vi "resonant.piezo.config.vi"() -> (3 "appended array":dbl[][](array[numeric]))   [LabVIEW 2012]
doc: "SciScan 1.2 160622"
uses:
  GFG/GFGnumericGet.vi
  GFG/GFGbooleanGet.vi
  GFG/GFG library.lvlib
panel:
  out "error out":errorcluster
  out "pockels cell control":dbl[](graph)
  out "piezo control":dbl[](graph)
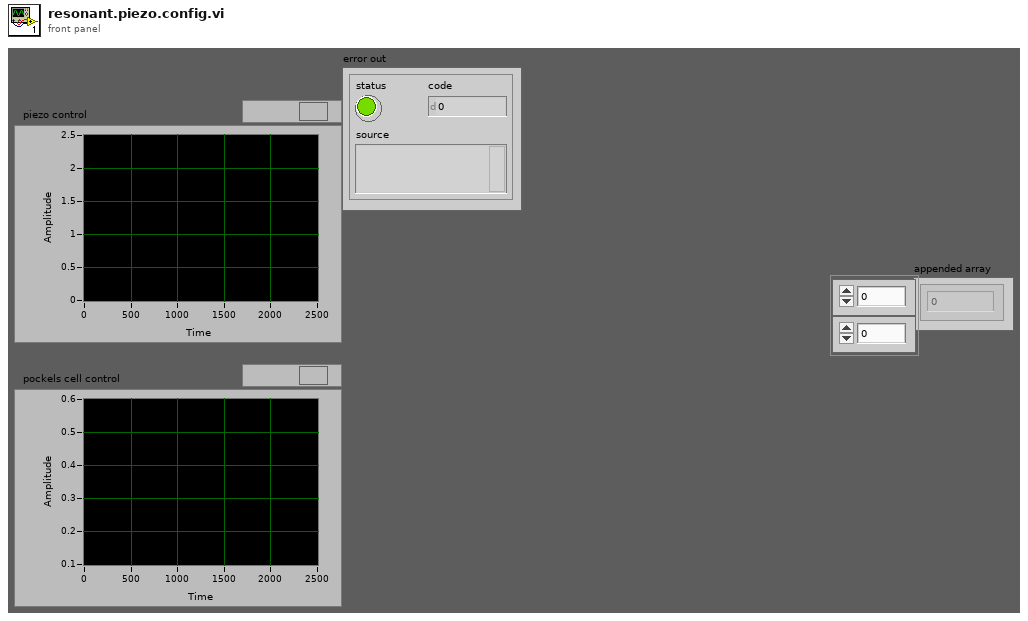
[diagram p1: front panel]
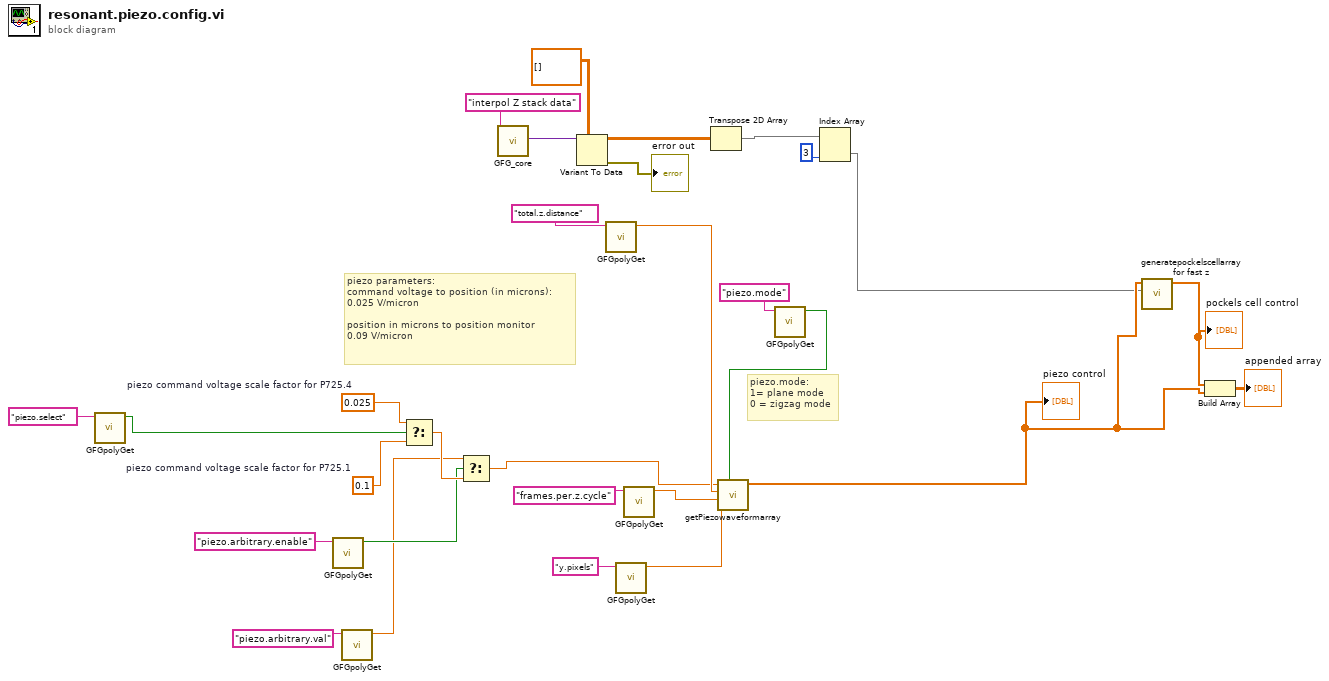
[diagram p0: block diagram]
diagram:
  w19 = 0.1  # piezo command voltage scale factor for P725.1
  w20 = 0.025  # piezo command voltage scale factor for P725.4
  # "piezo.mode: \n1= plane mode\n0 = zigzag mode"
  # "piezo parameters:\ncommand voltage to position (in microns):\n0.025 V/micron\n\nposition in microns to position monitor\n0.09 V/micron"
  n1 = call-poly "GFGpolyGet.vi"("Variable Name in"="piezo.select") -> ("Boolean Value OUT"=w17:bool)  [unwired: 9 in, 1 out]
  n2 = call-poly "GFGpolyGet.vi"("Variable Name in"="piezo.arbitrary.enable") -> ("Boolean Value OUT"=w3:bool)  [unwired: 9 in, 1 out]
  n3 = call-poly "GFGpolyGet.vi"("Variable Name in"="piezo.arbitrary.val" ("Tag in")) -> ("Numeric"=w2:dbl)  [unwired: 8 in, 2 out]
  n4 = Select(t=w20, s=w17, f=w19) -> (s? t:f=w4:dbl)
  n5 = Select(t=w2, s=w3, f=w4) -> (s? t:f=w1:dbl)
  n6 = call "GFG_core.vi"("Variable Name in"="interpol Z stack data") -> ("Variant Out"=w10:variant)  [unwired: 12 in, 6 out]
  n7 = Variant To Data(type=dbl[][] [] ("Interpolated Data"), Variant=w10) -> (data=w12:dbl[][], error out=→"error out":errorcluster)  [unwired: 1 in]
  n8 = call-poly "GFGpolyGet.vi"("Variable Name in"="total.z.distance") -> ("Numeric"=w8:dbl)  [unwired: 8 in, 2 out]
  n9 = call-poly "GFGpolyGet.vi"("Variable Name in"="y.pixels") -> ("Numeric"=w22:dbl)  [unwired: 8 in, 2 out]
  n10 = call-poly "GFGpolyGet.vi"("Variable Name in"="frames.per.z.cycle" ("Tag in")) -> ("Numeric"=w24:dbl)  [unwired: 8 in, 2 out]
  n11 = Transpose 2D Array(2D array=w12) -> (transposed array=w14:dbl[][])
  n12 = call-poly "GFGpolyGet.vi"("Variable Name in"="piezo.mode" ("Tag in")) -> ("Boolean Value OUT"=w27:bool)  [unwired: 9 in, 1 out]
  n13 = call "getPiezowaveformarray.vi"("sawtooth or zigzag"=w27, "pixel.num"=w22, "frames.per.z.cycle"=w24, "total.z.distance"=w8, "piezo scale factor"=w1) -> ("Array"=w23:dbl[])  [unwired: 6 in]
  "piezo control" <- w23
  n14 = Index Array(array=w14, index (col)=3 ("disabled index (col)")) -> (element=w9:dbl[])  [unwired: 1 in]
  n15 = call "generatepockelscellarray for fast z.vi"("interpolated pockels cell data"=w9, "piezo control"=w23) -> ("pockelscellarray"=w26:dbl[])  [unwired: 9 in]
  "pockels cell control" <- w26
  n16 = Build Array(w26, w23) -> (→"appended array":dbl[][])
